vi "Waypoint Monitor.vi"   [LabVIEW 2011]
uses:
  2 Globals/2 Global.vi
types:
  T1 = typedef "ocuWaypoints.ctl" = cluster{"Waypoints Array":cluster{"Point Type":u16, "Dist/Time":dbl, "UTM Location":T2}[], "Current Waypoint":dbl}
  T2 = typedef "UTM Location.ctl" = cluster{"UTM Zone":dbl, "Hemisphere":enum16{"North", "South"}, "East":dbl, "North":dbl}
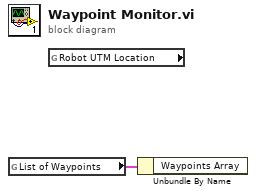
[diagram p0: block diagram]
diagram:
  n1 = global read "2 Global.vi" "List of Waypoints"() -> (w1:T1)
  n2 = global read "2 Global.vi" "Robot UTM Location"() -> ()  [unwired: 1 out]
  n3 = Unbundle By Name(w1) -> ()  [unwired: 1 out]
